vi "searchXMLNodes.vi"(8 "error in (no error)":errorcluster, 10 "XMLElement":string, 11 "xmlNode in":refnum<class "xmlNode.lvclass">) -> (0 "error out":errorcluster, 2 "xmlNodeArray":refnum<class "xmlNode.lvclass">[](array[class]), 3 "xmlNode out":refnum<class "xmlNode.lvclass">)   [LabVIEW 2011, in "Tools.lvlib" / "xml.lvlib" / "xmlNode.lvclass"]
uses:
  xmlNode.lvclass
  XmlParser.lvclass
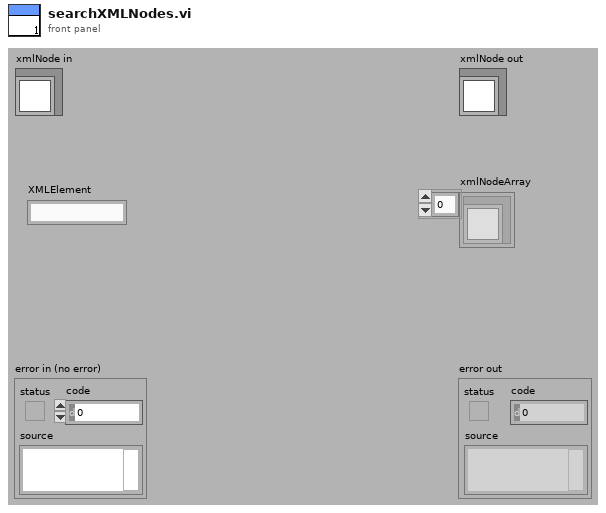
[diagram p1: front panel]
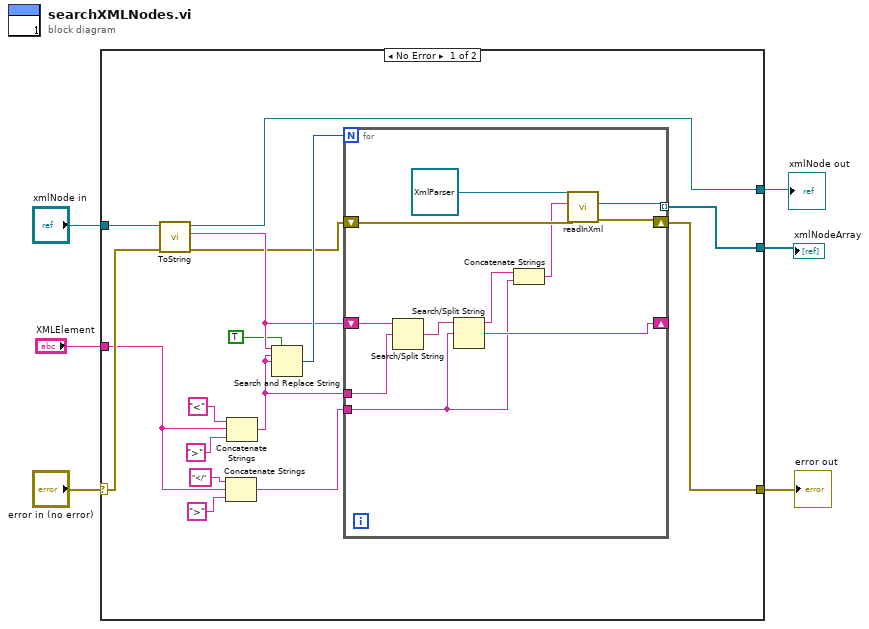
[diagram p0: block diagram]
diagram:
  n1 = case shown="No Error" "error in (no error)" {
    selector: "error in (no error)" -> [w21 w35]
    tunnel: [w7 w35] -> w5
    tunnel: [w15 w34] -> w3
    tunnel: "xmlNode in" -> [w22 w34]
    tunnel: "XMLElement" -> [w18 _]
    tunnel: [w8 _] -> w1
    frame No Error {
      n2 = call-dynamic "ToString.vi"("error in (no error)"=w21, "xmlNode in"=w22) -> ("error out"=w9:errorcluster, "xml"=w13:string, "xmlNode out"=w15:refnum<class "xmlNode.lvclass">)  [unwired: 7 in]
      n3 = Concatenate Strings("</", w18, ">") -> (w10:string)
      n4 = Concatenate Strings("<", w18, ">") -> (w11:string)
      n5 = Search and Replace String(replace all?=TRUE, input string=w13, search string=w11, replace string=w11) -> (number of replacements=w14:i32)  [unwired: 4 in, 3 out]
      n6 = for {
        N: w14 -> [_]
        tunnel: w11 -> [w30]
        shift-right: [w29] -> _
        shift-left: w13 -> [w31]
        tunnel: w10 -> [w28]
        tunnel: [w24] -> w8 mode=indexing
        shift-right: [w23] -> w7
        shift-left: w9 -> [w26]
        n7 = Search/Split String(string=w31, search string/char (-)=w30) -> (match + rest of string=w33:string)  [unwired: 1 in, 2 out]
        n8 = Search/Split String(string=w33, search string/char (-)=w28) -> (substring before match=w32:string, match + rest of string=w29:string)  [unwired: 1 in, 1 out]
        n9 = Concatenate Strings(w32, w28) -> (w25:string)
        n10 = call "readInXml.vi"("error in (no error)"=w26, "xmlString"=w25, "XmlParser in"=refnum<class "XmlParser.lvclass"> refnum ("Tools.lvlib:XmlParser.lvclass")) -> ("error out"=w23:errorcluster, "xmlNode"=w24:refnum<class "xmlNode.lvclass">)  [unwired: 6 in, 1 out]
      }
    }
    frame Error {
    }
  }
  "error out" <- w5
  "xmlNode out" <- w3
  "xmlNodeArray" <- w1
